vi "2D_Histogram.vi"(0 "X min":dbl, 1 "X max":dbl=10.0, 2 "X bins":i32=1000, 3 "Y min":dbl, 4 "Y max":dbl, 5 "Y bins":i32=1000, 6 "X":dbl[](array[numeric]), 7 "Y":dbl[](array[numeric])) -> (14 "X-Y 2-D Histogram":dbl[][](graph), 16 "Xoffset":dbl, 17 "Xmultiplier":dbl, 18 "Yoffset":dbl, 19 "Ymultiplier":dbl)   [LabVIEW 2009]
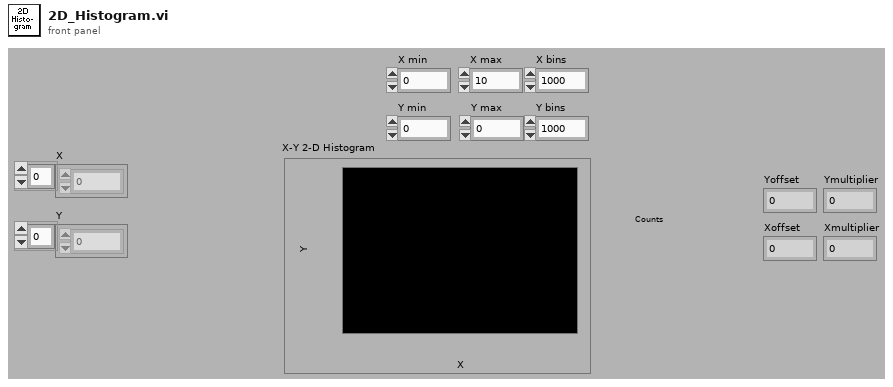
[diagram p1: front panel]
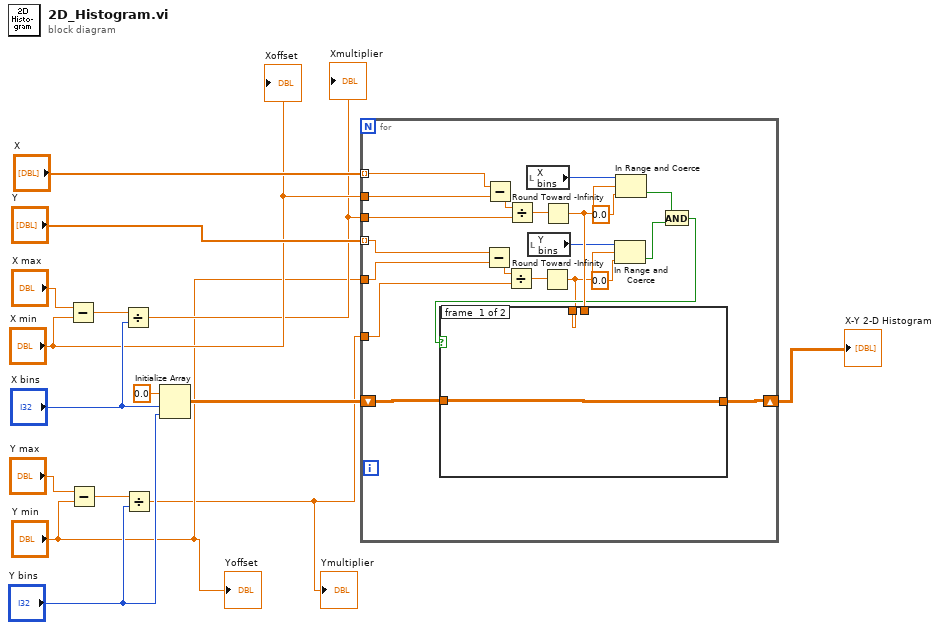
[diagram p0: block diagram]
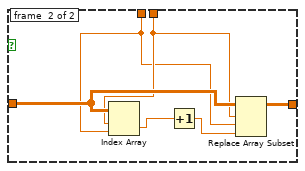
[diagram p2: hidden frame]
diagram:
  n1 = Subtract(x="X max", y="X min") -> (x-y=w12:dbl)
  n2 = Subtract(x="Y max", y="Y min") -> (x-y=w5:dbl)
  n3 = Divide(x=w12, y="X bins") -> (x/y=w6:dbl)
  "Xmultiplier" <- w6
  n4 = Divide(x=w5, y="Y bins") -> (x/y=w1:dbl)
  "Ymultiplier" <- w1
  n5 = Initialize Array(0.0 ("element"), "X bins", "Y bins") -> (w9:dbl[][])
  n6 = for {
    tunnel: "X" -> [w32] mode=indexing
    tunnel: "Y" -> [w31] mode=indexing
    tunnel: "Y min" -> [w30]
    tunnel: "X min" -> [w36]
    tunnel: w6 -> [w35]
    shift-right: [w33] -> w8
    shift-left: w9 -> [w34]
    tunnel: w1 -> [w29]
    n7 = Subtract(x=w31, y=w30) -> (x-y=w23:dbl)
    n8 = Subtract(x=w32, y=w36) -> (x-y=w28:dbl)
    n9 = Divide(x=w23, y=w29) -> (x/y=w22:dbl)
    n10 = Divide(x=w28, y=w35) -> (x/y=w27:dbl)
    n11 = local read "X bins"() -> (w26:i32)
    n12 = local read "Y bins"() -> (w20:i32)
    n13 = Round Toward -Infinity(1:w22) -> (0:w16:dbl)
    n14 = Round Toward -Infinity(1:w27) -> (0:w24:dbl)
    n15 = In Range and Coerce(upper limit=w20, x=w16, lower limit=0.0) -> (In Range?=w18:bool)  [unwired: 1 out]
    n16 = In Range and Coerce(upper limit=w26, x=w24, lower limit=0.0) -> (In Range?=w19:bool)  [unwired: 1 out]
    n17 = And(x=w19, y=w18) -> (x .and. y?=w17:bool)
    n18 = case shown="True" w17 {
      tunnel: w34 -> [w37 w42]
      tunnel: [w37 w40] -> w33
      tunnel: w24 -> [_ w39]
      tunnel: w16 -> [_ w38]
      frame #0 {
      }
      frame #1 {
        n19 = Index Array(array=w42, index (row)=w39, index (col)=w38) -> (element=w43:dbl)
        n20 = Increment(x=w43) -> (x+1=w41:dbl)
        n21 = Replace Array Subset(array=w42, new element=w41, index (row)=w39, index (col)=w38) -> (w40:dbl[][])
      }
    }
  }
  "X-Y 2-D Histogram" <- w8
  "Xoffset" <- "X min"
  "Yoffset" <- "Y min"
